vi "StartStopGen.vi"(9 "PlaneMode":T3 items=["XY Plane", "XZ Plane", "YZ Plane", "arbitraryplane"], 10 "AOLZ":dbl=0.0001 format="%#_13g", 11 "X-Y-Z coordinates":T2 {"Apparent Frame Size" format="%#_6f"; "Original FOV (um)" format="%#_6f"; "Pixels per miniscan" format="%#_6f"; "Dwell Time per pixel" format="%#_6f"; "Resolution" format="%#_6f"; "ROI group ID" format="%#_6f"; "Laser Power (%)" format="%#_6f"; "Zoom" format="%#_6f"; "Frame Size" format="%#_6f"; "Number of lines" format="%#_6f"; "Composite ID" format="%#_6f"; "Angle (deg)" format="%#_6f"; "ROI Time (ns)" format="%#_6f"; "ROI ID" format="%#_6f"; "Pixels in ROI" format="%#_6f"; "ROI index" format="%#_6f"; "Z stop" format="%#_6f"; "Y stop" format="%#_6f"; "X stop" format="%#_6f"; "Z start" format="%#_6f"; "X start" format="%#_6f"; "Y start" format="%#_6f"}) -> (3 "ROI Coordinates (broken down to miniscans)":T1)   [LabVIEW 2020]
uses:
  Typedefs/Plane Mode.ctl
  User Interface/Visualisation/Functional Imaging Viewer/Typedefs/ROI parameters data type.ctl
  Typedefs/ROI XY coordinates cluster.ctl
  Global Variables/gl_UI Ctrl Refs.vi
panel:
  out "Yc":dbl format="%#_13g"
  out "Xc":dbl format="%#_13g"
  out "anglearray":dbl[](array[numeric])
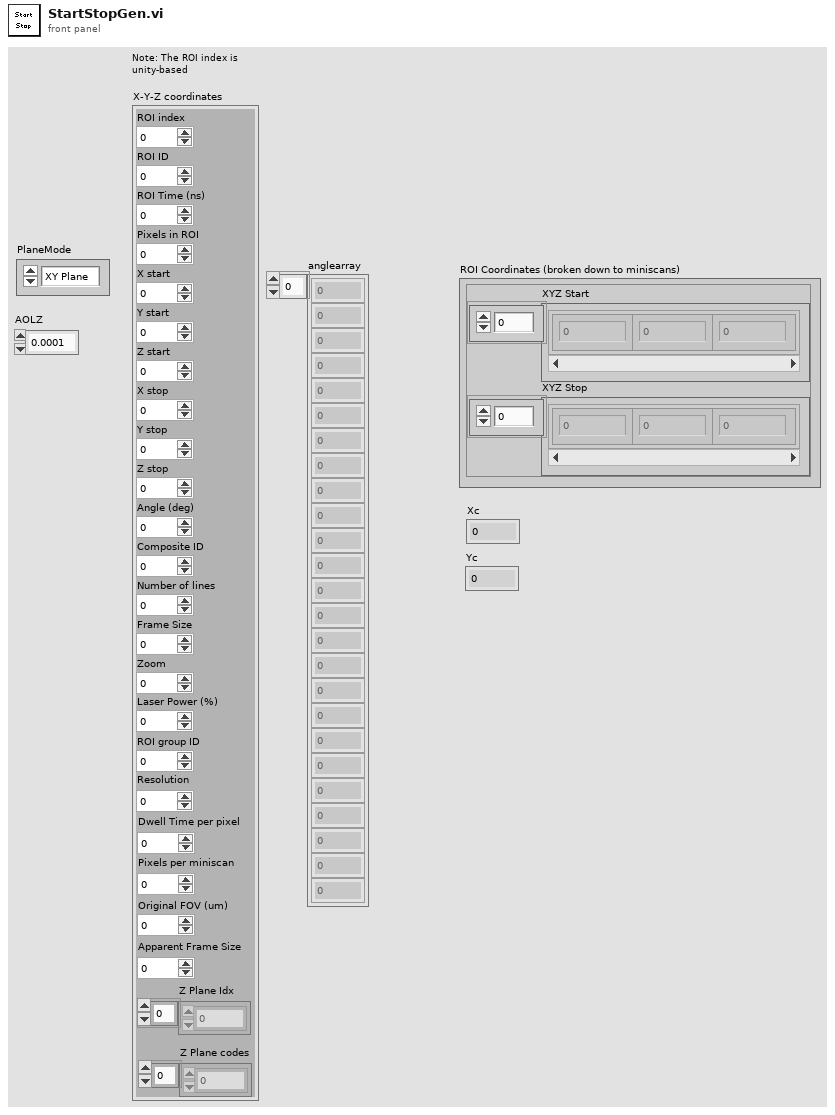
[diagram p1: front panel]
types:
  T1 = typedef "ROI XY coordinates cluster.ctl" = cluster{"XYZ Start":cluster{"X":sgl, "Y":sgl, "Z":sgl}[], "XYZ Stop":cluster{"X":sgl, "Y":sgl, "Z":sgl}[]}
  T2 = typedef "ROI parameters data type.ctl" = cluster{"ROI index":dbl, "ROI ID":dbl, "ROI Time (ns)":dbl, "Pixels in ROI":dbl, "X start":dbl, "Y start":dbl, "Z start":dbl, "X stop":dbl, "Y stop":dbl, "Z stop":dbl, "Angle (deg)":dbl, "Composite ID":dbl, "Number of lines":dbl, "Frame Size":dbl, "Zoom":dbl, "Laser Power (%)":dbl, "ROI group ID":dbl, "Resolution":dbl, "Dwell Time per pixel":dbl, "Pixels per miniscan":dbl, "Original FOV (um)":dbl, "Apparent Frame Size":dbl, "Z Plane Idx":i32[], "Z Plane codes":i32[]}
  T3 = typedef "Plane Mode.ctl" = u16
  T4 = typedef "UI ctrl refs cluster.ctl" = cluster{"Top level VI path":path, "Top level VI ref":refnum<vi>, "User menu ref":refnum<k9>, "Sub Panel control":refnum<vi>, "Imaging Param Tab":refnum<vi>, "Occurrence-Start drivers":refnum<k4>, "Occurrence-Speed logging initialised":refnum<k4>, "Occurrence-XYZ stage initialised":refnum<k4>, "Exit button":refnum<vi>, "Status ind":refnum<vi>, "Set as origin":refnum<vi>, "Speed Logging":refnum<vi>, "Time Lapse":refnum<vi>, "Live Imaging":refnum<vi>, "AOL Z Stack":refnum<vi>, "Motor Z Stack":refnum<vi>, "Funct Acq button":refnum<vi>, "Hard Shutter":refnum<vi>, "Virtual Shutter":refnum<vi>, "Laser Power":refnum<vi>, "AOL Mode":refnum<vi>, "Frame Size":refnum<vi>, "Field of View":refnum<vi>, "Dwell Time":refnum<vi>, "Zoom":refnum<vi>, "AOL Z":refnum<vi>, "Objective":refnum<vi>, "Axis":refnum<vi>, "Paths & Names":refnum<vi>, "Experiment folder path (ind.)":refnum<vi>, "Last State (Ind.)":refnum<vi>, "Averages":refnum<vi>, "Angle (degrees)":refnum<vi>, "X centre":refnum<vi>, "Y centre":refnum<vi>, "Plane Mode":refnum<vi>, "# Planes":refnum<vi>, "Z Start":refnum<vi>, "Z Stop":refnum<vi>, "Z Step":refnum<vi>, "PMT 1":refnum<vi>, "PMT 2":refnum<vi>, "Stage XYZ Position":refnum<vi>, "Pockels@Z Start":refnum<vi>, "Pockels@Z Stop":refnum<vi>, "Obtain Z Start":refnum<vi>, "Obtain Z Stop":refnum<vi>, "Live stim.trig.period":refnum<vi>, "Live stim.trig.enable":refnum<vi>, "Movement Correction":refnum<vi>, "Load Reference Image":refnum<vi>, "XY Stage Move":refnum<vi>, "MovCor Cluster":refnum<vi>, "RefDAQParam":refnum<vi>, "Funct. Acq. Pockels Modulation":refnum<vi>, "Ref Laser Power":refnum<vi>, "Enable Video Recording":refnum<vi>, "Video Record-Live Imaging":refnum<vi>, "Video Record-Funct acq":refnum<vi>, "Reference Source":refnum<vi>, "AOL Z-stack Chirps Ready (ind)":refnum<vi>, "Target time between mov.cor. ref triggers (ms)":refnum<vi>, "Funct. Acq. Ref frame save":refnum<vi>, "Tracking button":refnum<vi>, "Show ref plots window":refnum<vi>, "Center freq ind (nm)":refnum<vi>, "Pickup mode (ind)":refnum<vi>, "Logging queue (ind)":refnum<vi>, "Back aperture power (ind.)":refnum<vi>, "Power after objective (ind.)":refnum<vi>, "Switch user":refnum<vi>, "Ls1 Conn. Status":refnum<vi>, "Ls1Tuning Status":refnum<vi>, "Ls1 Faults":refnum<vi>, "Ls1 Connection":refnum<vi>, "Ls1 Mode":refnum<vi>, "Ls1 POWER [mW]":refnum<vi>, "Ls1Shutter":refnum<vi>, "Ls1 Wavelength":refnum<vi>, "Ls1 Note":refnum<vi>, "Ls1 Confirm Wav":refnum<vi>, "Ls1 PreChrp Prism1":refnum<vi>, "Ls1 PreChrp Prism2":refnum<vi>, "Ls1 wav top Ind":refnum<vi>, "Ls1 power top Ind":refnum<vi>, "Ls1 Pump peak Hold":refnum<vi>, "Ls1 Status Ind":refnum<vi>, "Ls1 wav cancel":refnum<vi>, "Experiment Type":refnum<vi>, "Biology Information":refnum<vi>, "Camera recording status":refnum<vi>}
  T5 = typedef "AOL_Globals.ctl" = cluster{"Imaging Protocol":T6, "Number of POI":u16, "Number of Miniscans":u16, "Number of Trials":u16, "Number of Cycles ":u64, "# Averaged Frames":u16, "Laser power (%)":u8, "Pockels (V)":dbl, "Acquisition Length (sec)":dbl, "Fill time (us)":dbl, "POI Dwell time (us)":dbl, "Miniscan Dwell time per pixel (us)":dbl, "PMT 1":dbl, "PMT 2":dbl, "Back Apperture (mA)":dbl, "Frame Size":T7, "Center Frequency":dbl, "Field of View (norm)":dbl, "DwellTime (us)":dbl, "Wavelength (nm)":dbl, "Zoom":dbl, "AOL Z":dbl, "AOL Mode":T8, "GridXY":dbl, "GridZ":dbl, "TriggerPeriod (sec)":dbl, "Number of Pixels in Miniscan":u16, "Experiment folder path":path, "X centre":dbl, "Y centre":dbl, "Angle (degrees)":dbl, "Plane Mode":T3, "Threshold":u16[], "Regenerate Chirps":bool, "Rectangle ROI length (pixels)":u16, "Rectangle ROI height (pixels)":u16, "AOD fill":u16, "StartupDelay":i32, "Samples Wait after Trigger":u16, "Slip Cycle":u32, "Add Cycle":bool, "Functional Mode":T9, "Z Start":dbl, "Z Stop":dbl, "# Planes":i32, "Total Pixels":i32, "Variable Miniscan Pixels":u16[], "Use Variable Length":bool, "Use Variable Resolution":bool, "Laser power (%) at Z Start":u8, "Laser power (%) at Z Stop":u8, "Ref Z Step":i8, "Ref Dwell Time (us)":dbl, "Field of View (um)":dbl}
  T6 = typedef "Imaging Protocols enum.ctl" = enum16{"AOL Z-Stack", "Motor Z Stack", "Functional Acquisition", "Single Plane Acquisition", "Volume Acquisition", "Live Imaging", "Live Plane Imaging", "Live Volume Imaging"}
  T7 = typedef "Frame Size.ctl" = u16
  T8 = typedef "AOL modes.ctl" = enum16{"Raster", "Structural", "Pointing", "Mini Scan", "Alignment"}
  T9 = typedef "Functional Mode.ctl" = enum16{"Point", "Line", "Patch", "Plane", "Volume"}
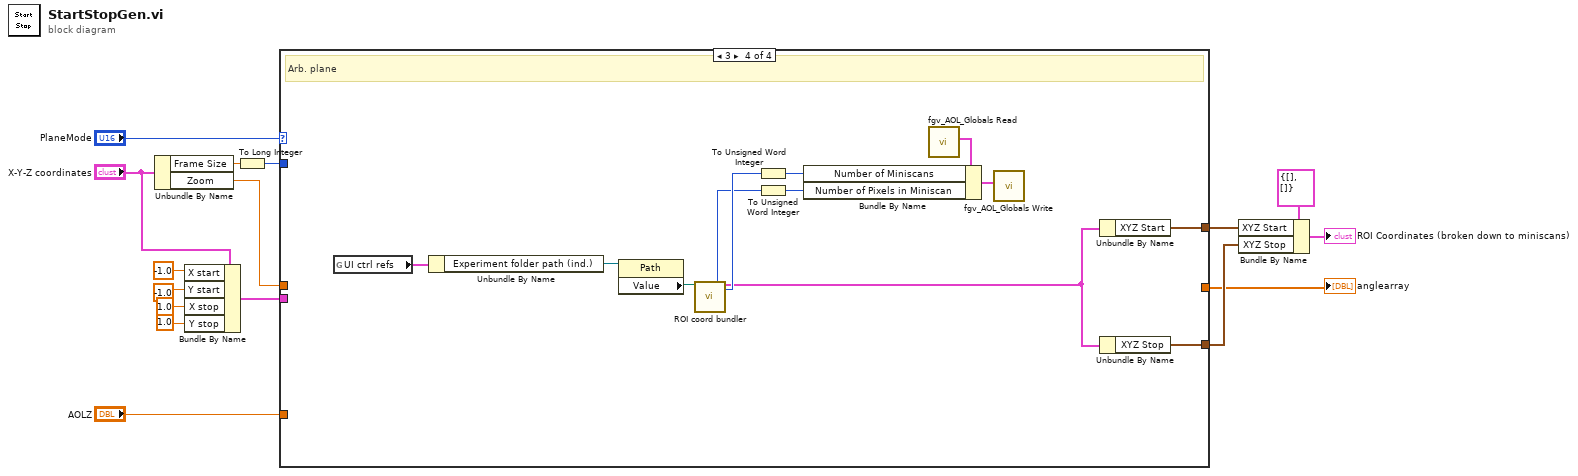
[diagram p0: block diagram]
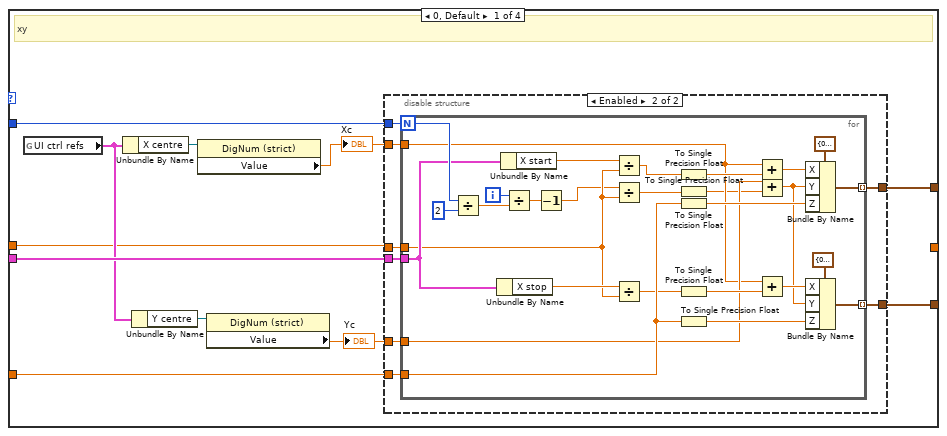
[diagram p2: hidden frame]
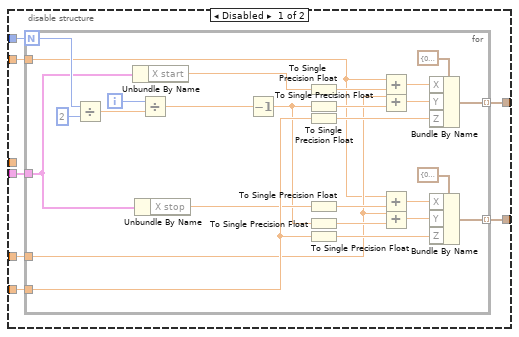
[diagram p3: hidden frame]
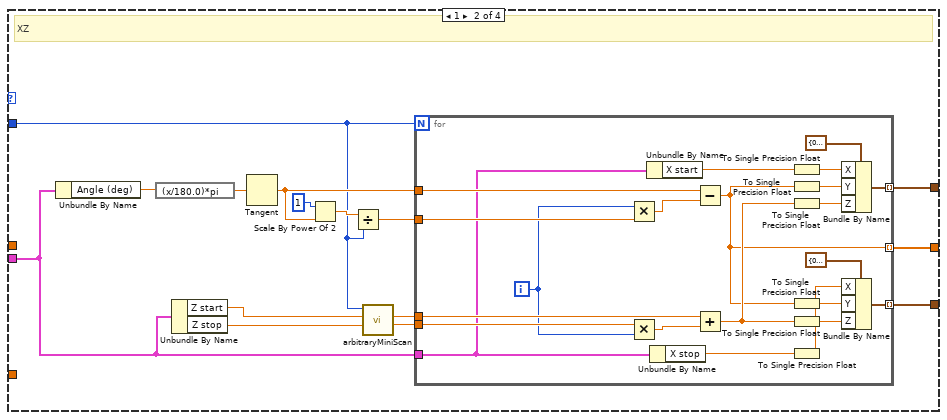
[diagram p4: hidden frame]
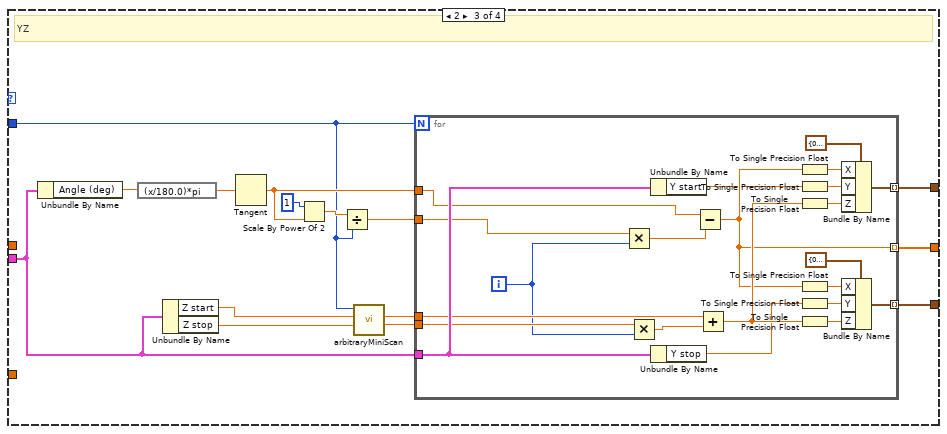
[diagram p5: hidden frame]
diagram:
  n1 = Unbundle By Name("X-Y-Z coordinates") -> ("Frame Size"=w10:dbl, "Zoom"=w1:dbl)
  n2 = Bundle By Name(cluster="X-Y-Z coordinates", "X start"=-1.0, "Y start"=-1.0 ("X start"), "X stop"=1.0, "Y stop"=1.0 ("X stop")) -> (w2:T2)
  n3 = To Long Integer(number=w10) -> (32bit integer=w14:i32)
  n4 = case shown="3" "PlaneMode" {
    tunnel: "AOLZ" -> [w27 _ _ _]
    tunnel: w14 -> [w26 w98 w135 _]
    tunnel: w2 -> [w23 w97 w134 _]
    tunnel: [w25 w110 w147 w171] -> w13
    tunnel: [w24 w111 w148 w179] -> w12
    tunnel: [_ w109 w146 _] -> w11
    tunnel: w1 -> [w17 _ _ _]
    frame 0, Default {
      # "xy"
      n5 = global read "gl_UI Ctrl Refs.vi" "UI ctrl refs"() -> (w18:T4)
      n6 = Unbundle By Name(w18) -> ("X centre"=w22:refnum<vi>)
      n7 = Unbundle By Name(w18) -> ("Y centre"=w20:refnum<vi>)
      n8 = property class="DigNum (strict)"(reference=w22) -> ("Value"=w21:dbl)  [unwired: 1 in, 2 out]
      "Xc" <- w21
      n9 = property class="DigNum (strict)"(reference=w20) -> ("Value"=w19:dbl)  [unwired: 1 in, 2 out]
      "Yc" <- w19
      n10 = disable-structure shown="Enabled" {
        disable-tunnel: w27 -> [w34 w68]
        disable-tunnel: w26 -> [w33 w67]
        disable-tunnel: [w32 w66] -> w25
        disable-tunnel: [w31 w65] -> w24
        disable-tunnel: w23 -> [w30 w64]
        disable-tunnel: w21 -> [w29 w63]
        disable-tunnel: w19 -> [w28 w62]
        disable-tunnel: w17 -> [_ w61]
        frame Disabled {
          n11 = for {
            N: w33 -> [w60]
            tunnel: w34 -> [w52]
            tunnel: w30 -> [w45]
            tunnel: [w50] -> w32 mode=indexing
            tunnel: [w49] -> w31 mode=indexing
            tunnel: w28 -> [w36]
            tunnel: w29 -> [w35]
            i -> [w56]
            n12 = Divide(x=w60, y=2) -> (x/y=w58:dbl)
            n13 = Unbundle By Name(w45) -> ("X start"=w47:dbl)
            n14 = Unbundle By Name(w45) -> ("X stop"=w48:dbl)
            n15 = Divide(x=w56, y=w58) -> (x/y=w57:dbl)
            n16 = Decrement(x=w57) -> (x-1=w46:dbl)
            n17 = To Single Precision Float(number=w47) -> (single precision float=w43:sgl)
            n18 = To Single Precision Float(number=w46) -> (single precision float=w41:sgl)
            n19 = To Single Precision Float(number=w52) -> (single precision float=w54:sgl)
            n20 = To Single Precision Float(number=w48) -> (single precision float=w40:sgl)
            n21 = To Single Precision Float(number=w46) -> (single precision float=w37:sgl)
            n22 = To Single Precision Float(number=w52) -> (single precision float=w53:sgl)
            n23 = Add(x=w35, y=w43) -> (x+y=w44:dbl)
            n24 = Add(x=w36, y=w41) -> (x+y=w42:dbl)
            n25 = Add(x=w35, y=w40) -> (x+y=w39:dbl)
            n26 = Add(x=w36, y=w37) -> (x+y=w38:dbl)
            n27 = Bundle By Name(cluster=cluster{"X":sgl, "Y":sgl, "Z":sgl} {"X"=0.0, "Y"=0.0, "Z"=0.0} ("XYZ"), "X"=w44, "Y"=w42, "Z"=w54) -> (w49:cluster{"X":sgl, "Y":sgl, "Z":sgl})
            n28 = Bundle By Name(cluster=cluster{"X":sgl, "Y":sgl, "Z":sgl} {"X"=0.0, "Y"=0.0, "Z"=0.0} ("XYZ"), "X"=w39, "Y"=w38, "Z"=w53) -> (w50:cluster{"X":sgl, "Y":sgl, "Z":sgl})
          }
        }
        frame Enabled {
          n29 = for {
            N: w67 -> [w96]
            tunnel: w68 -> [w89]
            tunnel: w64 -> [w85]
            tunnel: [w87] -> w66 mode=indexing
            tunnel: [w86] -> w65 mode=indexing
            tunnel: w62 -> [w80]
            tunnel: w63 -> [w79]
            tunnel: w61 -> [w73]
            i -> [w93]
            n30 = Divide(x=w96, y=2) -> (x/y=w94:dbl)
            n31 = Unbundle By Name(w85) -> ("X stop"=w75:dbl)
            n32 = Unbundle By Name(w85) -> ("X start"=w78:dbl)
            n33 = Divide(x=w93, y=w94) -> (x/y=w70:dbl)
            n34 = Decrement(x=w70) -> (x-1=w69:dbl)
            n35 = Divide(x=w78, y=w73) -> (x/y=w77:dbl)
            n36 = Divide(x=w69, y=w73) -> (x/y=w76:dbl)
            n37 = Divide(x=w75, y=w73) -> (x/y=w74:dbl)
            n38 = To Single Precision Float(number=w77) -> (single precision float=w83:sgl)
            n39 = To Single Precision Float(number=w76) -> (single precision float=w72:sgl)
            n40 = To Single Precision Float(number=w89) -> (single precision float=w91:sgl)
            n41 = To Single Precision Float(number=w74) -> (single precision float=w82:sgl)
            n42 = To Single Precision Float(number=w89) -> (single precision float=w90:sgl)
            n43 = Add(x=w79, y=w83) -> (x+y=w84:dbl)
            n44 = Add(x=w80, y=w72) -> (x+y=w71:dbl)
            n45 = Add(x=w79, y=w82) -> (x+y=w81:dbl)
            n46 = Bundle By Name(cluster=cluster{"X":sgl, "Y":sgl, "Z":sgl} {"X"=0.0, "Y"=0.0, "Z"=0.0} ("XYZ"), "X"=w84, "Y"=w71, "Z"=w91) -> (w86:cluster{"X":sgl, "Y":sgl, "Z":sgl})
            n47 = Bundle By Name(cluster=cluster{"X":sgl, "Y":sgl, "Z":sgl} {"X"=0.0, "Y"=0.0, "Z"=0.0} ("XYZ"), "X"=w81, "Y"=w71, "Z"=w90) -> (w87:cluster{"X":sgl, "Y":sgl, "Z":sgl})
          }
        }
      }
    }
    frame 1 {
      # "XZ"
      n48 = Unbundle By Name(w97) -> ("Angle (deg)"=w108:dbl)
      n49 = expression code="(x/180.0)*pi" ("degrees to radians")(w108) -> (w105:dbl)
      n50 = Unbundle By Name(w97) -> ("Z start"=w101:dbl, "Z stop"=w102:dbl)
      n51 = Tangent(1:w105) -> (0:w104:dbl)
      n52 = Scale By Power Of 2(n=i16 1, x=w104) -> (x*2^n=w107:dbl)
      n53 = Divide(x=w107, y=w98) -> (x/y=w103:dbl)
      n54 = call "arbitraryMiniScan.vi"("Norm zStop in"=w102, "Norm zStart"=w101, "FrameSize"=w98) -> ("StepSize"=w99:dbl, "min_coordinate"=w100:dbl)  [unwired: 7 in]
      n55 = for {
        N: w98 -> [_]
        tunnel: w99 -> [w133]
        tunnel: w100 -> [w131]
        tunnel: w103 -> [w130]
        tunnel: [w118] -> w111 mode=indexing
        tunnel: [w117] -> w110 mode=indexing
        tunnel: [w116] -> w109 mode=indexing
        tunnel: w104 -> [w115]
        tunnel: w97 -> [w112]
        i -> [w128]
        n56 = Multiply(x=w128, y=w130) -> (x*y=w129:dbl)
        n57 = Multiply(x=w133, y=w128) -> (x*y=w132:dbl)
        n58 = Unbundle By Name(w112) -> ("X start"=w113:dbl)
        n59 = Unbundle By Name(w112) -> ("X stop"=w114:dbl)
        n60 = Subtract(x=w115, y=w129) -> (x-y=w116:dbl)
        n61 = Add(x=w131, y=w132) -> (x+y=w119:dbl)
        n62 = To Single Precision Float(number=w113) -> (single precision float=w126:sgl)
        n63 = To Single Precision Float(number=w116) -> (single precision float=w125:sgl)
        n64 = To Single Precision Float(number=w119) -> (single precision float=w124:sgl)
        n65 = To Single Precision Float(number=w116) -> (single precision float=w122:sgl)
        n66 = To Single Precision Float(number=w119) -> (single precision float=w121:sgl)
        n67 = To Single Precision Float(number=w114) -> (single precision float=w123:sgl)
        n68 = Bundle By Name(cluster=cluster{"X":sgl, "Y":sgl, "Z":sgl} {"X"=0.0, "Y"=0.0, "Z"=0.0} ("XYZ"), "X"=w126, "Y"=w125, "Z"=w124) -> (w118:cluster{"X":sgl, "Y":sgl, "Z":sgl})
        n69 = Bundle By Name(cluster=cluster{"X":sgl, "Y":sgl, "Z":sgl} {"X"=0.0, "Y"=0.0, "Z"=0.0} ("XYZ"), "X"=w123, "Y"=w122, "Z"=w121) -> (w117:cluster{"X":sgl, "Y":sgl, "Z":sgl})
      }
    }
    frame 2 {
      # "YZ"
      n70 = Unbundle By Name(w134) -> ("Angle (deg)"=w145:dbl)
      n71 = expression code="(x/180.0)*pi" ("degrees to radians")(w145) -> (w142:dbl)
      n72 = Unbundle By Name(w134) -> ("Z start"=w138:dbl, "Z stop"=w139:dbl)
      n73 = Tangent(1:w142) -> (0:w141:dbl)
      n74 = Scale By Power Of 2(n=i16 1, x=w141) -> (x*2^n=w144:dbl)
      n75 = Divide(x=w144, y=w135) -> (x/y=w140:dbl)
      n76 = call "arbitraryMiniScan.vi"("Norm zStop in"=w139, "Norm zStart"=w138, "FrameSize"=w135) -> ("StepSize"=w136:dbl, "min_coordinate"=w137:dbl)  [unwired: 7 in]
      n77 = for {
        N: w135 -> [_]
        tunnel: w134 -> [w170]
        tunnel: w136 -> [w169]
        tunnel: w137 -> [w167]
        tunnel: w140 -> [w165]
        tunnel: w141 -> [w149]
        tunnel: [w154] -> w148 mode=indexing
        tunnel: [w153] -> w147 mode=indexing
        tunnel: [w152] -> w146 mode=indexing
        i -> [w166]
        n78 = Multiply(x=w165, y=w166) -> (x*y=w164:dbl)
        n79 = Multiply(x=w169, y=w166) -> (x*y=w168:dbl)
        n80 = Unbundle By Name(w170) -> ("Y start"=w150:dbl)
        n81 = Unbundle By Name(w170) -> ("Y stop"=w151:dbl)
        n82 = Subtract(x=w149, y=w164) -> (x-y=w152:dbl)
        n83 = Add(x=w167, y=w168) -> (x+y=w155:dbl)
        n84 = To Single Precision Float(number=w152) -> (single precision float=w162:sgl)
        n85 = To Single Precision Float(number=w150) -> (single precision float=w161:sgl)
        n86 = To Single Precision Float(number=w155) -> (single precision float=w160:sgl)
        n87 = To Single Precision Float(number=w152) -> (single precision float=w159:sgl)
        n88 = To Single Precision Float(number=w151) -> (single precision float=w158:sgl)
        n89 = To Single Precision Float(number=w155) -> (single precision float=w157:sgl)
        n90 = Bundle By Name(cluster=cluster{"X":sgl, "Y":sgl, "Z":sgl} {"X"=0.0, "Y"=0.0, "Z"=0.0} ("XYZ"), "X"=w162, "Y"=w161, "Z"=w160) -> (w154:cluster{"X":sgl, "Y":sgl, "Z":sgl})
        n91 = Bundle By Name(cluster=cluster{"X":sgl, "Y":sgl, "Z":sgl} {"X"=0.0, "Y"=0.0, "Z"=0.0} ("XYZ"), "X"=w159, "Y"=w158, "Z"=w157) -> (w153:cluster{"X":sgl, "Y":sgl, "Z":sgl})
      }
    }
    frame 3 {
      # "Arb. plane"
      n92 = global read "gl_UI Ctrl Refs.vi" "UI ctrl refs"() -> (w182:T4)
      n93 = Unbundle By Name(w182) -> ("Experiment folder path (ind.)"=w181:refnum<vi>)
      n94 = property class="Path"(reference=w181) -> ("Value"=w180:path)  [unwired: 1 in, 2 out]
      n95 = call "ROI coord bundler.vi"("Experiment folder path"=w180) -> ("Number of pixels in single miniscan"=w175:i32, "ROI Coordinates (broken down to miniscans)"=w172:T1, "Total number of miniscans"=w176:i32)  [unwired: 8 in, 8 out]
      n96 = To Unsigned Word Integer(number=w176) -> (unsigned 16bit integer=w174:u16)
      n97 = To Unsigned Word Integer(number=w175) -> (unsigned 16bit integer=w173:u16)
      n98 = call "fgv_AOL_Globals Read.vi"() -> ("AOL_Globals"=w178:T5)  [unwired: 9 in, 2 out]
      n99 = Bundle By Name(cluster=w178, "Number of Miniscans"=w174, "Number of Pixels in Miniscan"=w173) -> (w177:T5)
      n100 = call "fgv_AOL_Globals Write.vi"("AOL_Globals"=w177) -> ()  [unwired: 10 in, 1 out]
      n101 = Unbundle By Name(w172) -> ("XYZ Start"=w179:cluster{"X":sgl, "Y":sgl, "Z":sgl}[])
      n102 = Unbundle By Name(w172) -> ("XYZ Stop"=w171:cluster{"X":sgl, "Y":sgl, "Z":sgl}[])
    }
  }
  "anglearray" <- w11
  n103 = Bundle By Name(cluster=T1 {"XYZ Start"=[], "XYZ Stop"=[]} ("ROI Coordinates (broken down to miniscans)"), "XYZ Start"=w12, "XYZ Stop"=w13) -> (→"ROI Coordinates (broken down to miniscans)":T1)
